vi "stop_sweep.vi"(8 "error in (no error)":errorcluster, 11 "ImagingModeDL090130Frame in":refnum<class "ImagingModeDL090130Frame.lvclass">=refnum) -> (0 "error out":errorcluster, 3 "ImagingModeDL090130Frame out":refnum<class "ImagingModeDL090130Frame.lvclass">)   [LabVIEW 2010, in "ImagingModeDL090130Frame.lvclass"]
uses:
  ImagingModeDL090130Frame.lvclass
  ImagingModeDL090130Frame.lvclass/ImagingModeDL090130Frame.ctl
  common/xcontrols/XIntensityCompensation/XIntensityCompensation/XIntensityCompensation.xctl
  ImagingModeDL090923Scaffold/ImagingModeDL090923Scaffold/ImagingModeDL090923Scaffold.lvclass
  common/classes/GenericComponent/GenericComponent/class_data.vi
  common/classes/ErrorController/ErrorController/class_data.vi
  common/classes/ErrorController/ErrorController/ErrorController.lvclass
  common/classes/GenericComponent/GenericComponent/GenericComponent.lvclass
  Stage/GenericStage/GenericStage/trigger_enum.ctl
  Stage/GenericStage/GenericStage/GenericStage.lvclass
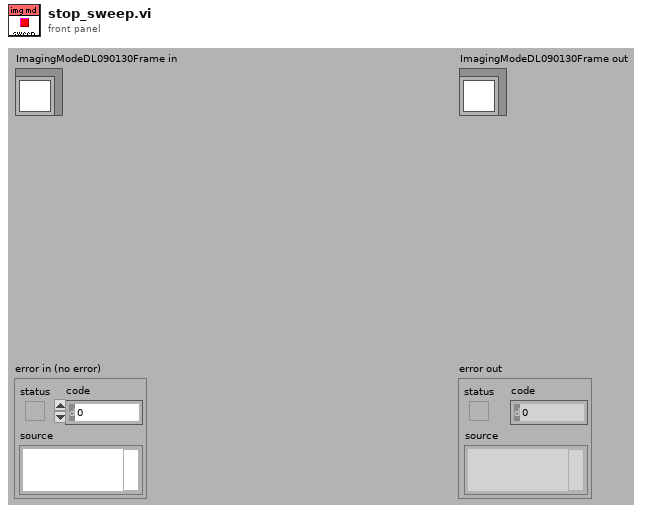
[diagram p1: front panel]
types:
  T1 = typedef "GenericStage.lvclass/trigger_enum.ctl" = enum16{"NULL", "move", "update position", "set origin", "return to origin"}
  T2 = typedef "ImagingModeDL090130Frame.lvclass/control_refs.ctl" = cluster{"resolution controls":cluster{"x pixels":refnum<vi>, "y pixels":refnum<vi>, "ratio x factor":refnum<vi>, "ratio y factor":refnum<vi>}, "speed controls":cluster{"pixel dwell time":refnum<vi>, "line scan time":refnum<vi>, "frame rate":refnum<vi>}, "number of frames controls":cluster{"# of frames":refnum<vi>, "duration":refnum<vi>, "# of repetitions":refnum<vi>}, "current value indicators":cluster{"frame #":refnum<vi>, "repetition #":refnum<vi>, "offset":refnum<vi>}, "step controls":cluster{"step size":refnum<vi>, "return to origin?":refnum<vi>, "translation mode":refnum<vi>, "XIntensityCompensation":refnum<vi>}, "settings":refnum<vi>, "defineButton":refnum<vi>}
  T3 = typedef "ImagingModeDL090130Frame.lvclass/translation_mode_enum.ctl" = enum16{"scanHead", "stage"}
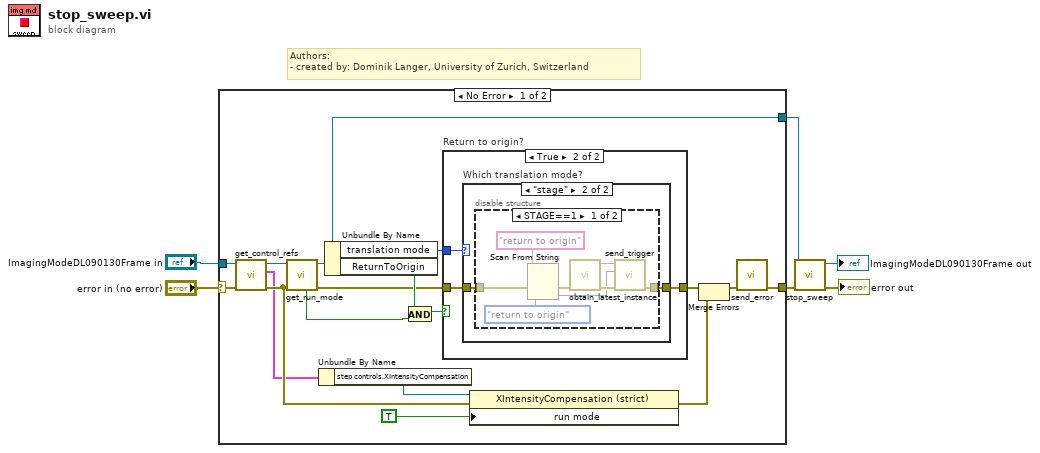
[diagram p0: block diagram]
diagram:
  # "Authors: \n- created by: Dominik Langer, University of Zurich, Switzerland"
  n1 = case shown="No Error" "error in (no error)" {
    selector: "error in (no error)" -> [w14 w41]
    tunnel: [w18 w41] -> w3
    tunnel: [w19 w40] -> w1
    tunnel: "ImagingModeDL090130Frame in" -> [w16 w40]
    frame No Error {
      n2 = call-dynamic "get_control_refs.vi"("error in (no error)"=w14, "ImagingModeDL090130Frame in"=w16) -> ("error out"=w13:errorcluster, "control refs"=w12:T2, "ImagingModeDL090130Frame out"=w15:refnum<class "ImagingModeDL090130Frame.lvclass">)  [unwired: 7 in]
      n3 = call "get_run_mode.vi"("error in (no error)"=w13, "GenericPlugin in"=w15) -> ("error out"=w21:errorcluster, "GenericPlugin out"=w19:refnum<class "ImagingModeDL090130Frame.lvclass">, "is NOT free run?"=w20:bool)  [unwired: 5 in, 2 out]
      n4 = Unbundle By Name(w12) -> ("step controls.XIntensityCompensation"=w17:refnum<vi>)
      n5 = Unbundle By Name(w19) -> ("translation mode"=w7:T3, "ReturnToOrigin"=w23:bool)
      n6 = And(x=w23, y=w20) -> (x .and. y?=w22:bool)
      n7 = case "Return to origin?" shown="True" w22 {
        tunnel: w21 -> [w24 w27]
        tunnel: [w24 w26] -> w8
        tunnel: w7 -> [_ w25]
        frame False {
        }
        frame True {
          n8 = case "Which translation mode?" shown="\"stage\"" w25 {
            tunnel: w27 -> [w28 w30]
            tunnel: [w28 w29] -> w26
            frame "scanHead", Default {
            }
            frame "stage" {
              n9 = disable-structure shown="STAGE==1" {
                disable-tunnel: w30 -> [w35 w39]
                disable-tunnel: [w37 w39] -> w29
                frame condition #0 {
                  n10 = Scan From String(input string="return to origin", error in=w35, default 1=trigger_enum."return to origin" ("trigger")) -> (error out=w34:errorcluster, output 1=w32:T1)  [unwired: 2 in, 2 out]
                  n11 = call "obtain_latest_instance.vi"("error in (no error)"=w34) -> ("error out"=w38:errorcluster, "GenericStage out"=w36:refnum<class "GenericStage.lvclass">)  [unwired: 9 in]
                  n12 = call-dynamic "send_trigger.vi"("error in (no error)"=w38, "trigger"=w32, "GenericStage in"=w36) -> ("error out"=w37:errorcluster)  [unwired: 7 in, 1 out]
                }
                frame condition #1 (active) {
                }
              }
            }
          }
        }
      }
      n13 = property class="XIntensityCompensation (strict)"(reference=w17, error in=w13, "run mode"=TRUE ("free-run mode")) -> (error out=w10:errorcluster)  [unwired: 1 out]
      n14 = Merge Errors(w8, w10) -> (w9:errorcluster)
      n15 = call "send_error.vi"("error in (no error)"=w9) -> ("error out"=w18:errorcluster)  [unwired: 10 in]
    }
    frame Error {
    }
  }
  n16 = call-parent "stop_sweep.vi"("error in (no error)"=w3, "ScanModeDL090923Scaffold in"=w1) -> ("error out"=→"error out":errorcluster, "ScanModeDL090923Scaffold out"=→"ImagingModeDL090130Frame out":refnum<class "ImagingModeDL090130Frame.lvclass">)  [unwired: 8 in]
